vi "Verify Parameterized.vi"(8 "error in (no error)":errorcluster, 9 "Set (map: control name  -> value as variant)":set{map{string, variant}}(c389), 10 "VI in":refnum<vi>) -> (0 "error out":errorcluster, 1 "Failure Message":string, 2 "Passed?":bool)   [LabVIEW 2020, in "Approval Tests.lvlib"]
uses:
  Approval Tests.lvlib
  <vilib>/JDP Science/JSONtext/JSONtext.lvlib
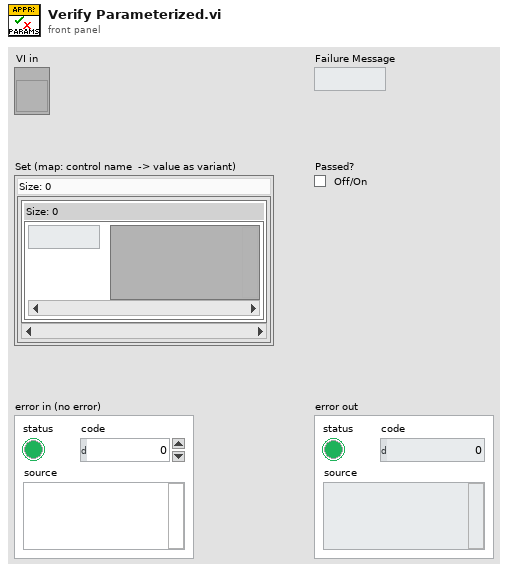
[diagram p1: front panel]
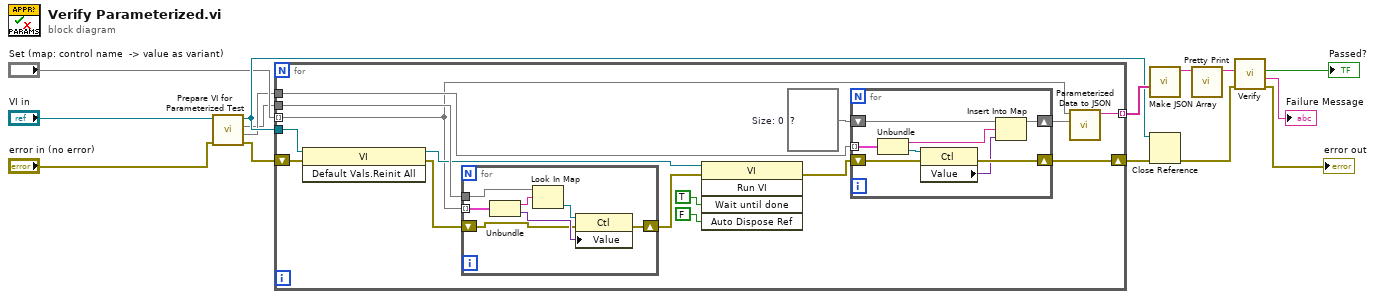
[diagram p0: block diagram]
diagram:
  n1 = call "Prepare VI for Parameterized Test.vi"("error in (no error)"="error in (no error)", "VI in"="VI in") -> ("error out"=w3:errorcluster, "Indicators"=w2:map{string, refnum<vi>}, "Controls"=w1:map{string, refnum<vi>}, "VI out"=w9:refnum<vi>)  [unwired: 6 in]
  n2 = for {
    tunnel: w1 -> [w27]
    tunnel: w2 -> [w26]
    tunnel: w9 -> [w24]
    tunnel: [w18] -> w10 mode=indexing
    tunnel: "Set (map: control name  -> value as variant)" -> [w19] mode=indexing
    shift-right: [w20] -> w5
    shift-left: w3 -> [w21]
    w17 = map{string, variant} {}  # Size: 0
    n3 = invoke on="Invoke Node" class="VI" method="Default Vals.Reinit All"(reference=w24, error in=w21) -> (reference out=w23:refnum<vi>, error out=w25:errorcluster)  [unwired: 1 in, 1 out]
    n4 = for {
      tunnel: w27 -> [w45]
      tunnel: w19 -> [w44] mode=indexing
      shift-right: [w40] -> w28
      shift-left: w25 -> [w39]
      n5 = Unbundle(w44) -> ("key"=w43:string, "Variant"=w41:variant)
      n6 = Look In Map(map=w45, key=w43) -> (value=w42:refnum<vi>)  [unwired: 1 in, 1 out]
      n7 = property on="Property Node" class="Ctl"(reference=w42, error in=w39, "Value"=w41) -> (error out=w40:errorcluster)  [unwired: 1 out]
    }
    n8 = invoke on="Invoke Node" class="VI" method="Run VI"(reference=w23, error in=w28, "Wait until done"=TRUE ("Wait Until Done"), "Auto Dispose Ref"=FALSE ("Auto Dispose Reference")) -> (error out=w22:errorcluster)  [unwired: 1 in, 4 out]
    n9 = for {
      tunnel: w26 -> [w38] mode=indexing
      shift-right: [w35] -> w20
      shift-left: w22 -> [w36]
      shift-right: [w32] -> w16
      shift-left: w17 -> [w31]
      n10 = Unbundle(w38) -> (w34:string, "reference"=w37:refnum<vi>)
      n11 = property on="Property Node" class="Ctl"(reference=w37, error in=w36) -> (error out=w35:errorcluster, "Value"=w33:variant)  [unwired: 1 out]
      n12 = Insert Into Map(map in=w31, key=w34, value=w33) -> (map out=w32:map{string, variant})  [unwired: 2 out]
    }
    n13 = call "Parameterized Data to JSON.vi"("Outputs"=w16, "Inputs"=w19) -> ("<JSON>"=w18:string)  [unwired: 9 in]
  }
  n14 = call <vilib>:"Make JSON Array.vi"("JSON Elements"=w10) -> ("<JSON>"=w11:string)  [unwired: 9 in, 1 out]
  n15 = Close Reference(reference=w9, error in (no error)=w5) -> (error out=w8:errorcluster)
  n16 = call <vilib>:"Pretty Print.vi"("JSON"=w11) -> ("<JSON>"=w13:string)  [unwired: 8 in, 2 out]
  n17 = call "Verify.vi"("error in"=w8, "Anything"=w13) -> ("error out"=→"error out":errorcluster, "Failure Message"=→"Failure Message":string, "Passed?"=→"Passed?":bool)  [unwired: 7 in]
